vi "_setRef.vi"(7 "parentURL":string, 8 "error in (no error)":errorcluster, 9 "Name":string, 10 "Refnum":variant, 11 "TagDB in":T1) -> (0 "error out":errorcluster, 2 "URL":string, 3 "TagDB out":T1)   [LabVIEW 2017, in "TagDB RefManager.lvlib"]
uses:
  TagDB RefManager.lvlib
  <userlib>/_NEVSTOP/TagDB/Typedef/TagDB.ctl
  <vilib>/Utility/Data Type/Type Definitions/Refnum Type.ctl
  <vilib>/Utility/Data Type/Type Definitions/VI Server Generic Type.ctl
  <vilib>/Utility/Data Type/NI_Data Type.lvlib
  <userlib>/_NEVSTOP/TagDB/TagDB.lvlib
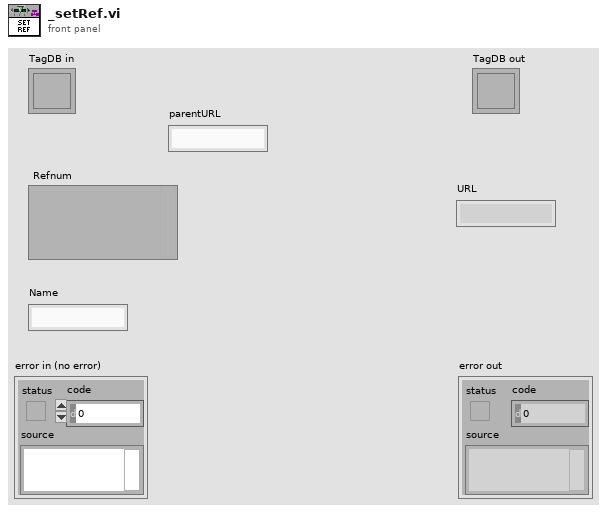
[diagram p1: front panel]
types:
  T1 = typedef "TagDB.lvlib/TagDB.ctl" = refnum<k1>
  T2 = typedef "NI_Data Type.lvlib/Data Type.ctl" = enum8{"Invalid Type", "Void", "I8", "I16", "I32", "I64", "U8", "U16", "U32", "U64", "Single Float", "Double Float", "Extended Float", "Single Complex", "Double Complex", "Extended Complex", "Enum U8", "Enum U16", "Enum U32", "Enum U64", "Single Float With Unit", "Double Float With Unit", "Extended Float With Unit", "Single Complex with Unit", "Double Complex with Unit", "Extended Complex with Unit", "Boolean", "String", "Path", "Picture", "Tag", "Array", "Cluster", "Variant", "LV Variant", "Waveform", "Timestamp", "Digital Waveform", "Digital Data", "ExpressData", "Refnum", "External Data", "VI", "Poly VI", "LabVIEW Class Instance", "Fixed Point"}
  T3 = typedef "NI_Data Type.lvlib/Refnum Type.ctl" = enum16{"NotARefnum", "UnknownRefnum", "Generic", "Datalog", "ByteStream", "Device", "Occurence", "TCPNetConnection", "Auto", "Menu", "Imaq", "Hardware", "DataSocket", "Visa", "IVI", "UDPNetConnection", "Notifier", "Queue", "Irda", "EventReg", "DotNet", "UserEvent", "Callback", "UNUSED_EMPTY_POSITION", "BlueToothNetConnection", "LVObjApp", "LVObjVI", "LVObjUnknown", "GenericClass", "UserDefinedRefnumTag", "DataValue", "RT FIFO", "TDMS File"}
  T4 = typedef "NI_Data Type.lvlib/VI Server Generic Type.ctl" = enum16{"NoType", "\tkLVObjApp=0x1", "\tkLVObjVI", "\tkLVObjGeneric", "\tkLVObjDecoration", "\tkLVObjText", "\tkLVObjControl", "\tkLVObjColorBox", "\tkLVObjBoolean", "\tkLVObjRefNum", "\tkLVObjVariant", "\tkLVObjPath", "\tkLVObjListBox", "\tkLVObjTable", "\tkLVObjArray", "\tkLVObjPicture", "\tkLVObjOleContainer", "\tkLVObjNumeric", "\tkLVObjDigital", "\tkLVObjNamedNumeric", "\tkLVObjColorRamp", "\tkLVObjSlide", "\tkLVObjGraphOrChart", "\tkLVObjWaveformChart", "\tkLVObjWaveformGraph", "\tkLVObjIntensityChart", "\tkLVObjIntensityGraph", "\tkLVObjString", "\tkLVObjIOName", "\tkLVObjComboBox", "\tkLVObjCluster", "\tkLVObjPanel", "\tkLVObjKnob", "\tkLVObjNumWithScale", "\tkLVObjRing", "\tkLVObjEnum", "\tkLVObjGObject", "\tkLVObjPlot", "\tkLVObjCursor", "\tkLVObjNumericText", "\tkLVObjScale", "\tkLVObjColorScale", "\tkLVObjGraphScale", "\tkLVObjColorGraphScale", "\tkLVObjTypedRefNum", "\tkLVObjOldKnobScale", "\tkLVObjMCListbox", "\tkLVObjMeasureData", "\tkLVObjDSCTag", "\tkLVObjDAQName", "\tkLVObjVISAName", "\tkLVObjIVIName", "\tkLVObjSlideScale", "\tkLVObjTabControl", "\tkLVObjPage", "\tkLVObjTabArrayTabControl", "\tkLVObjConPane", "\tkLVObjDAQMXName", "\tkLVObjVIRefNum", "\tkLVObjLVObjRefNum", "\tkLVObjAbsTime", "\tkLVObjDigitalTable", "\tkLVObjUnused", "\tkLVObjUnused2", "\tkLVObjSCLControl", "\tkLVObjSubPanel", "\tkLVObjTreeControl", "\tkLVObjGenClassTagRef", "\tkLVObjGenClassRef", "\tkLVObjRotaryColorScale", "\tkLVObjPlugInDDOControl", "\tkLVObjPlugInDDOClassHolder", "\tkLVObjRadClusControl", "\tkLVObjProject", "\tkLVObjProjectItem", "\tkLVObjPane", "\tkLVObjSplitterBar", "\tkLVObjProjectBuildItem", "\tkLVObjPixmap", "\tkLVObjFacadeVI", "\tkLVObjLibrary", "\tkLVObjVariable", "\tkLVObjPropertyBag", "\tkLVObjXYGraph", "\tkLVObjScene", "\tkLVObjUDClassLibrary", "\tkLVObjUDClassClone", "\tkLVObjMethodVI", "\tkLVObjXCtlLibrary", "\tkLVObjXNodeLibrary", "\tkLVObjScroll", "\tkLVObjLVTarget", "\tkLVObjMixedGraph", "\tkLVObjProvider", "\tkLVObjCopyOperation", "\tkLVObjTargetItem", "\tkLVObjProjectItemType", "\tkLVObjCopyItem", "\tkLVObjCopyConflict", "\tkLVObjCopyExpert", "\tkLVObjSceneGraphDisp", "\tkLVObjPolyVI", "\tkLVObjLVClassDDO", "kLVObjDiagram=0x4000", "\tkLVObjTerminal", "\tkLVObjConstant", "\tkLVObjPathConstant", "\tkLVObjArrayConstant", "\tkLVObjNumericConstant", "\tkLVObjDigitalNumConstant", "\tkLVObjNamedNumericConstant", "\tkLVObjStringConstant", "\tkLVObjClusterConstant", "\tkLVObjFixedConstant", "\tkLVObjControlTerminal", "\tkLVObjFormulaParameter", "\tkLVObjGlobal", "\tkLVObjLocal", "\tkLVObjRightShiftRegister", "\tkLVObjFunction", "\tkLVObjSubVI", "\tkLVObjCallByRef", "\tkLVObjUnitCast", "\tkLVObjStructure", "\tkLVObjLoop", "\tkLVObjMultiframeStructure", "\tkLVObjSequence", "\tkLVObjCaseSelector", "\tkLVObjFormula", "\tkLVObjGrowableFunction", "\tkLVObjBuildClusterArray", "\tkLVObjCompoundArithmetic", "\tkLVObjIndexArray", "\tkLVObjBuildArray", "\tkLVObjNamedBundler", "\tkLVObjCIN", "\tkLVObjCallLibrary", "\tkLVObjObjectFunction", "\tkLVObjProperty", "\tkLVObjInvoke", "\tkLVObjNode", "\tkLVObjBooleanConstant", "\tkLVObjBlockDiagram", "\tkLVObjRingConstant", "\tkLVObjEnumConstant", "\tkLVObjTunnel", "\tkLVObjLoopTunnel", "\tkLVObjSequenceLocal", "\tkLVObjComparison", "\tkLVObjReadWriteFile", "\tkLVObjTypeCast", "\tkLVObjFlattenUnflattenString", "\tkLVObjGPIBReadWrite", "\tkLVObjForLoop", "\tkLVObjWhileLoop", "\tkLVObjScriptNode", "\tkLVObjArrayToCluster", "\tkLVObjFormatScanString", "\tkLVObjWire", "\tkLVObjProbe", "\tkLVObjInnerTerminal", "\tkLVObjLeftShiftRegister", "\tkLVObjPolySubVI", "\tkLVObjPropItem", "\tkLVObjIONameConstant", "\tkLVObjDSCTagConstant", "\tkLVObjDAQNameConstant", "\tkLVObjVISANameConstant", "\tkLVObjIVINameConstant", "\tkLVObjColorBoxConstant", "\tkLVObjControlRefConstant", "\tkLVObjClassSpecifierConstant", "\tkLVObjConfNode", "\tkLVObjMasterWizard", "\tkLVObjStateDiagWizard", "\tkLVObjOuterTerminal", "\tkLVObjDAQMXNameConstant", "\tkLVObjEventStructure", "\tkLVObjFlatSequence", "\tkLVObjGenClassTagRefConstant", "\tkLVObjAbsTimeConstant", "\tkLVObjExternalNode", "\tkLVObjSubWizard", "\tkLVObjScriptNodeParameter", "\tkLVObjStatVIRef", "\tkLVObjComboBoxConstant", "\tkLVObjTimedLoop", "\tkLVObjGenClassDeepCopy", "\tkLVObjGenClassTagFlat", "\tkLVObjGenClassTagFlatRefConstant", "\tkLVObjGenClassFlat", "\tkLVObjSimDiagram", "\tkLVObjCompDiagram", "\tkLVObjSimNode", "\tkLVObjSimDCO", "\tkLVObjBundler", "\tkLVObjUnbundler", "\tkLVObjNamedUnbundler", "\tkLVObjFlatSeqFrame", "\tkLVObjFlatSeqInTun", "\tkLVObjFlatSeqOutTun", "\tkLVObjRefNumConst", "\tkLVObjFlattenString", "\tkLVObjPolySelector", "\tkLVObjXNode", "\tkLVObjSelectorTunnel", "\tkLVObjCommentNode", "\tkLVObjSdfDiagram", "\tkLVObjSDFCompDiagram", "\tkLVObjSdfNode", "\tkLVObjSdfDCO", "\tkLVObjFileDialog", "\tkLVObjTLDCO", "\tkLVObjTimeSeqFrame", "\tkLVObjTimeFlatSequence", "\tkLVObjTimedSequence", "\tkLVObjXDataNode", "\tkLVObjCodeWizard", "\tkLVObjMathScriptNode", "\tkLVObjMathScriptNodeParameter", "\tkLVObjLVClassBDConst"}
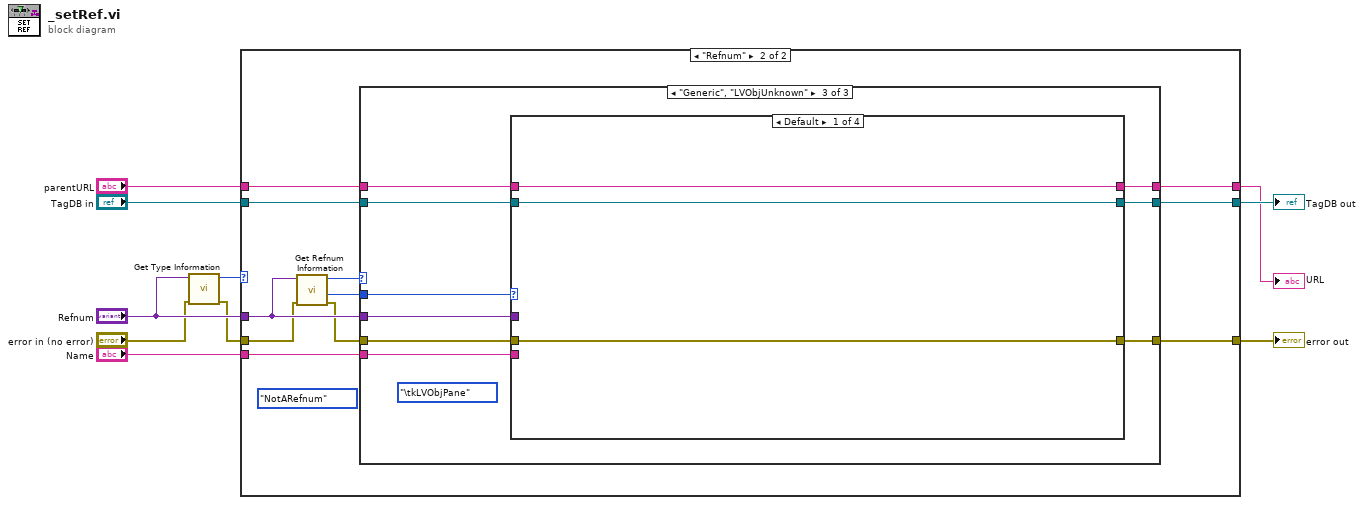
[diagram p0: block diagram]
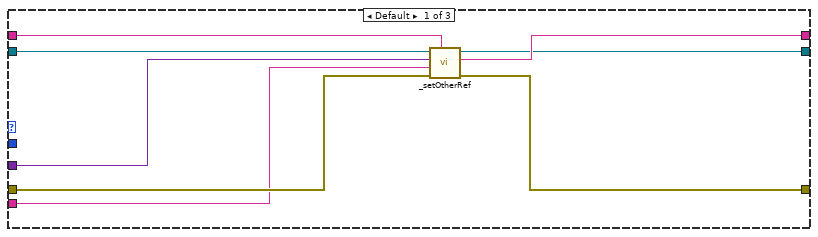
[diagram p3: hidden frame]
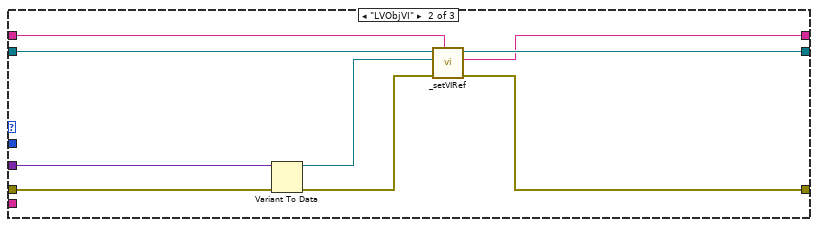
[diagram p4: hidden frame]
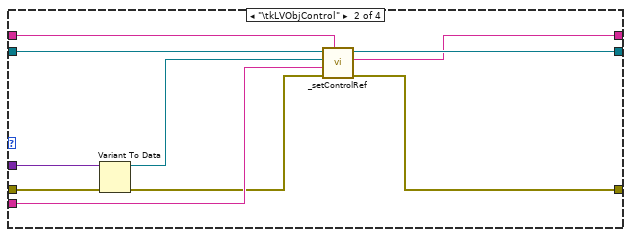
[diagram p5: hidden frame]
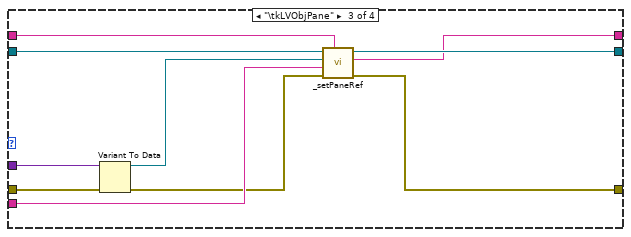
[diagram p6: hidden frame]
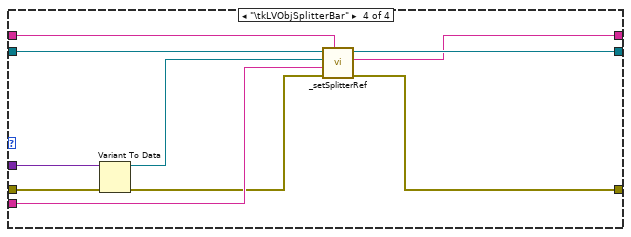
[diagram p7: hidden frame]
diagram:
  n1 = call <vilib>:"Get Type Information.vi"("error in (no error)"="error in (no error)", "Variant"="Refnum") -> ("error out"=w1:errorcluster, "Type"=w10:T2)  [unwired: 5 in, 3 out]
  n2 = case shown="\"Refnum\"" w10 {
    tunnel: [w13 w24] -> w9
    tunnel: "TagDB in" -> [w13 w23]
    tunnel: [w12 w22] -> w7
    tunnel: w1 -> [w12 w17]
    tunnel: "Refnum" -> [_ w21]
    tunnel: "parentURL" -> [w11 w20]
    tunnel: "Name" -> [_ w19]
    tunnel: [w11 w18] -> w3
    frame Default {
    }
    frame "Refnum" {
      (unwired) Refnum_Type."NotARefnum" ("Reference Type")
      n3 = call <vilib>:"Get Refnum Information.vi"("error in (no error)"=w17, "Variant"=w21) -> ("error out"=w16:errorcluster, "VI Server Generic Type"=w14:T4, "Reference Type"=w15:T3)  [unwired: 6 in, 1 out]
      n4 = case shown="\"Generic\", \"LVObjUnknown\"" w15 {
        tunnel: [w30 w39 w48] -> w24
        tunnel: w23 -> [w29 w41 w50]
        tunnel: [w28 w38 w47] -> w22
        tunnel: w16 -> [w27 w35 w44]
        tunnel: w20 -> [w32 w40 w49]
        tunnel: w19 -> [w26 _ w46]
        tunnel: w21 -> [w25 w37 w45]
        tunnel: [w31 w33 w43] -> w18
        tunnel: w14 -> [_ _ w42]
        frame Default {
          n5 = call "_setOtherRef.vi"("parentURL"=w32, "error in (no error)"=w27, "Name"=w26, "Refnum"=w25, "TagDB in"=w29) -> ("error out"=w28:errorcluster, "Ref-Key"=w31:string, "TagDB out"=w30:T1)  [unwired: 4 in]
        }
        frame "LVObjVI" {
          n6 = Variant To Data(error in=w35, Variant=w37) -> (data=w36:refnum<vi>, error out=w34:errorcluster)  [unwired: 1 in]
          n7 = call "_setVIRef.vi"("parentURL"=w40, "error in (no error)"=w34, "Refnum"=w36, "TagDB in"=w41) -> ("error out"=w38:errorcluster, "URL"=w33:string, "TagDB out"=w39:T1)  [unwired: 5 in]
        }
        frame "Generic", "LVObjUnknown" {
          (unwired) VI_Server_Generic_Type."\tkLVObjPane" ("VI Server Generic Type")
          n8 = case shown="Default" w42 {
            tunnel: w50 -> [w52 w63 w73 w83]
            tunnel: w49 -> [w53 w62 w72 w82]
            tunnel: [w52 w61 w71 w81] -> w48
            tunnel: [w51 w60 w70 w80] -> w47
            tunnel: w46 -> [_ w59 w69 w79]
            tunnel: w45 -> [_ w58 w68 w78]
            tunnel: w44 -> [w51 w57 w67 w77]
            tunnel: [w53 w55 w65 w75] -> w43
            frame Default {
            }
            frame "\tkLVObjControl" {
              n9 = Variant To Data(error in=w57, Variant=w58) -> (data=w54:refnum<vi>, error out=w56:errorcluster)  [unwired: 1 in]
              n10 = call "_setControlRef.vi"("parentURL"=w62, "error in (no error)"=w56, "Name"=w59, "Refnum"=w54, "TagDB in"=w63) -> ("error out"=w60:errorcluster, "Ref-Key"=w55:string, "TagDB out"=w61:T1)  [unwired: 4 in]
            }
            frame "\tkLVObjPane" {
              n11 = Variant To Data(error in=w67, Variant=w68) -> (data=w64:refnum<vi>, error out=w66:errorcluster)  [unwired: 1 in]
              n12 = call "_setPaneRef.vi"("parentURL"=w72, "error in (no error)"=w66, "Name"=w69, "Refnum"=w64, "TagDB in"=w73) -> ("error out"=w70:errorcluster, "URL"=w65:string, "TagDB out"=w71:T1)  [unwired: 4 in]
            }
            frame "\tkLVObjSplitterBar" {
              n13 = Variant To Data(error in=w77, Variant=w78) -> (data=w74:refnum<vi>, error out=w76:errorcluster)  [unwired: 1 in]
              n14 = call "_setSplitterRef.vi"("parentURL"=w82, "error in (no error)"=w76, "Name"=w79, "Refnum"=w74, "TagDB in"=w83) -> ("error out"=w80:errorcluster, "URL"=w75:string, "TagDB out"=w81:T1)  [unwired: 4 in]
            }
          }
        }
      }
    }
  }
  "error out" <- w7
  "TagDB out" <- w9
  "URL" <- w3
